vi "Fetch Measurements.vi"(8 "error in (no error)":errorcluster, 11 "Scope In":refnum<k15>) -> (0 "error out":errorcluster, 1 "Phase":dbl format="%.2f", 2 "Actual Gain":dbl, 3 "Scope out":refnum<k15>, 5 "wfm":waveform(dbl)[](array[waveform]))   [LabVIEW 2023, in "Bode Plot - PXI.lvlib"]
uses:
  Bode Plot - PXI.lvlib
  <instrlib>/niScope/Controls/niScope timestamp type.ctl
  <instrlib>/niScope/Controls/niScope scalar measurement.ctl
  <instrlib>/niScope/Controls/niScope array measurement.ctl
  <instrlib>/niScope/Controls/niScope clearable measurement.ctl
  <instrlib>/niScope/Acquire/niScope Multi Read WDT.vi
  <instrlib>/niScope/Measurements/niScope Fetch Measurement.vi
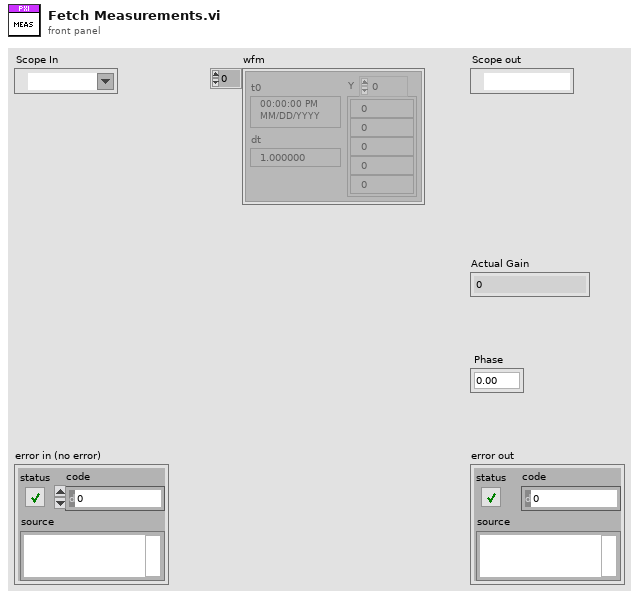
[diagram p1: front panel]
types:
  T1 = typedef "niScope clearable measurement.ctl" = i32
  T2 = typedef "niScope array measurement.ctl" = i32
  T3 = typedef "niScope scalar measurement.ctl" = i32
  T4 = typedef "niScope timestamp type.ctl" = i32
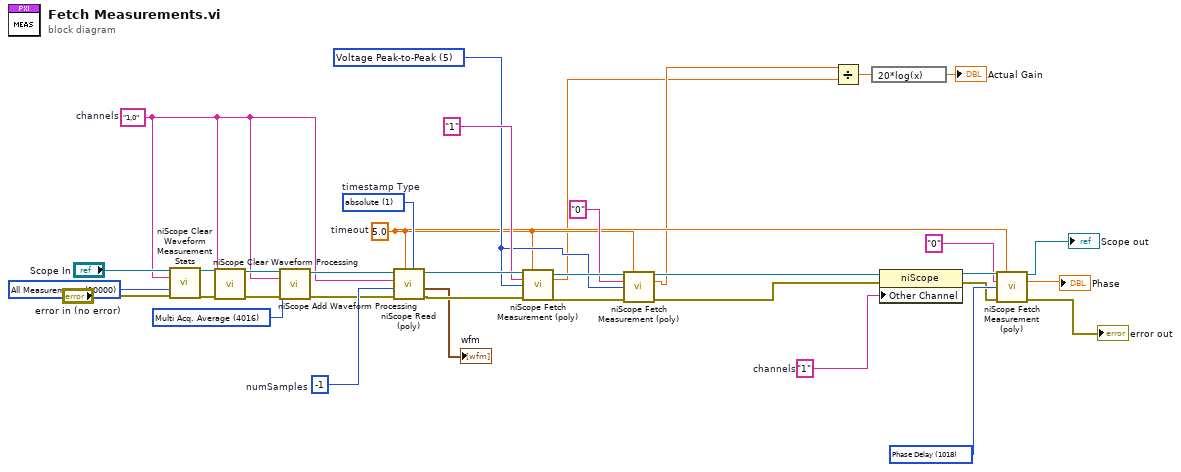
[diagram p0: block diagram]
diagram:
  w5 = T1 10000 items=["All Measurements"=10000, "Multi Acq. Voltage Histogram"=4004, "Multi Acq. Time Histogram"=4005, "Multi Acq. Average"=4016, "Frequency"=2, "Average Frequency"=1016, "FFT Frequency"=1008, "Period"=3, "Average Period"=1015, "Rise Time"=0, "Fall Time"=1, "Rising Slew Rate"=1010, "Falling Slew Rate"=1011, "Overshoot"=18, "Preshoot"=19, "Voltage RMS"=4, "Voltage Cycle RMS"=16, "AC Estimate"=1012, "FFT Amplitude"=1009, "Voltage Average"=10, "Voltage Cycle Average"=17, "DC Estimate"=1013, "Voltage Max"=6, "Voltage Min"=7, "Voltage Peak-to-Peak"=5, "Voltage High"=8, "Voltage Low"=9, "Voltage Amplitude"=15, "Voltage Top"=1007, "Voltage Base"=1006, "Voltage Base-to-Top"=1017, "Negative Width"=11, "Positive Width"=12, "Negative Duty Cycle"=13, "Positive Duty Cycle"=14, "Integral"=1005, "Area"=1003, "Cycle Area"=1004, "Time Delay"=1014, "Phase Delay"=1018, "Low Ref Volts"=1000, "Mid Ref Volts"=1001, "High Ref Volts"=1002, "Volt. Hist. Mean"=2000, "Volt. Hist. Stdev"=2001, "Volt. Hist. Median"=2003, "Volt. Hist. Mode"=2010, "Volt. Hist. Max"=2005, "Volt. Hist. Min"=2006, "Volt. Hist. Peak-to-Peak"=2002, "Volt. Hist. Mean + Stdev"=2007, "Volt. Hist. Mean + 2 Stdev"=2008, "Volt. Hist. Mean + 3 Stdev"=2009, "Volt. Hist. Hits"=2004, "Volt. Hist. New Hits"=2011, "Time Hist. Mean"=3000, "Time Hist. Stdev"=3001, "Time Hist. Median"=3003, "Time Hist. Mode"=3010, "Time Hist. Max"=3005, "Time Hist. Min"=3006, "Time Hist. Peak-to-Peak"=3002, "Time Hist. Mean + Stdev"=3007, "Time Hist. Mean + 2 Stdev"=3008, "Time Hist. Mean + 3 Stdev"=3009, "Time Hist. Hits"=3004, "Time Hist. New Hits"=3011] ("clearable measurement")
  w21 = T2 4016 items=["None"=4000, "Last Acq. Histogram"=4001, "Multi Acq. Voltage Histogram"=4004, "Multi Acq. Time Histogram"=4005, "Multi Acq. Average"=4016, "Polynomial Interpolation"=4011, "Array Integral"=4006, "Derivative"=4007, "Inverse"=4008, "Multiply Channels"=4012, "Add Channels"=4013, "Subtract Channels"=4014, "Divide Channels"=4015, "Array Offset"=4025, "Array Gain"=4026, "Hanning Window"=4009, "Flat Top Window"=4010, "Hamming Window"=4020, "Triangle Window"=4023, "Blackman Window"=4024, "FIR Windowed Filter"=4021, "Bessel IIR Filter"=4022, "Butterworth IIR Filter"=4017, "Chebyshev IIR Filter"=4018, "FFT Phase Spectrum"=4002, "FFT Amp. Spectrum (Volts RMS)"=4003, "FFT Amp. Spectrum (dB)"=4019] ("array measurement")
  w1 = "1,0"  # channels
  w31 = "1"  # channels
  w33 = T3 1018 items=["None"=4000, "Frequency"=2, "Average Frequency"=1016, "FFT Frequency"=1008, "Period"=3, "Average Period"=1015, "Rise Time"=0, "Fall Time"=1, "Rising Slew Rate"=1010, "Falling Slew Rate"=1011, "Overshoot"=18, "Preshoot"=19, "Voltage RMS"=4, "Voltage Cycle RMS"=16, "AC Estimate"=1012, "FFT Amplitude"=1009, "Voltage Average"=10, "Voltage Cycle Average"=17, "DC Estimate"=1013, "Voltage Max"=6, "Voltage Min"=7, "Voltage Peak-to-Peak"=5, "Voltage High"=8, "Voltage Low"=9, "Voltage Amplitude"=15, "Voltage Top"=1007, "Voltage Base"=1006, "Voltage Base-to-Top"=1017, "Negative Width"=11, "Positive Width"=12, "Negative Duty Cycle"=13, "Positive Duty Cycle"=14, "Integral"=1005, "Area"=1003, "Cycle Area"=1004, "Time Delay"=1014, "Phase Delay"=1018, "Low Ref Volts"=1000, "Mid Ref Volts"=1001, "High Ref Volts"=1002, "Volt. Hist. Mean"=2000, "Volt. Hist. Stdev"=2001, "Volt. Hist. Median"=2003, "Volt. Hist. Mode"=2010, "Volt. Hist. Max"=2005, "Volt. Hist. Min"=2006, "Volt. Hist. Peak-to-Peak"=2002, "Volt. Hist. Mean + Stdev"=2007, "Volt. Hist. Mean + 2 Stdev"=2008, "Volt. Hist. Mean + 3 Stdev"=2009, "Volt. Hist. Hits"=2004, "Volt. Hist. New Hits"=2011, "Time Hist. Mean"=3000, "Time Hist. Stdev"=3001, "Time Hist. Median"=3003, "Time Hist. Mode"=3010, "Time Hist. Max"=3005, "Time Hist. Min"=3006, "Time Hist. Peak-to-Peak"=3002, "Time Hist. Mean + Stdev"=3007, "Time Hist. Mean + 2 Stdev"=3008, "Time Hist. Mean + 3 Stdev"=3009, "Time Hist. Hits"=3004, "Time Hist. New Hits"=3011] ("scalar measurement")
  w13 = T3 5 items=["None"=4000, "Frequency"=2, "Average Frequency"=1016, "FFT Frequency"=1008, "Period"=3, "Average Period"=1015, "Rise Time"=0, "Fall Time"=1, "Rising Slew Rate"=1010, "Falling Slew Rate"=1011, "Overshoot"=18, "Preshoot"=19, "Voltage RMS"=4, "Voltage Cycle RMS"=16, "AC Estimate"=1012, "FFT Amplitude"=1009, "Voltage Average"=10, "Voltage Cycle Average"=17, "DC Estimate"=1013, "Voltage Max"=6, "Voltage Min"=7, "Voltage Peak-to-Peak"=5, "Voltage High"=8, "Voltage Low"=9, "Voltage Amplitude"=15, "Voltage Top"=1007, "Voltage Base"=1006, "Voltage Base-to-Top"=1017, "Negative Width"=11, "Positive Width"=12, "Negative Duty Cycle"=13, "Positive Duty Cycle"=14, "Integral"=1005, "Area"=1003, "Cycle Area"=1004, "Time Delay"=1014, "Phase Delay"=1018, "Low Ref Volts"=1000, "Mid Ref Volts"=1001, "High Ref Volts"=1002, "Volt. Hist. Mean"=2000, "Volt. Hist. Stdev"=2001, "Volt. Hist. Median"=2003, "Volt. Hist. Mode"=2010, "Volt. Hist. Max"=2005, "Volt. Hist. Min"=2006, "Volt. Hist. Peak-to-Peak"=2002, "Volt. Hist. Mean + Stdev"=2007, "Volt. Hist. Mean + 2 Stdev"=2008, "Volt. Hist. Mean + 3 Stdev"=2009, "Volt. Hist. Hits"=2004, "Volt. Hist. New Hits"=2011, "Time Hist. Mean"=3000, "Time Hist. Stdev"=3001, "Time Hist. Median"=3003, "Time Hist. Mode"=3010, "Time Hist. Max"=3005, "Time Hist. Min"=3006, "Time Hist. Peak-to-Peak"=3002, "Time Hist. Mean + Stdev"=3007, "Time Hist. Mean + 2 Stdev"=3008, "Time Hist. Mean + 3 Stdev"=3009, "Time Hist. Hits"=3004, "Time Hist. New Hits"=3011] ("scalar measurement")
  w35 = T4 1 items=["relative", "absolute"]  # timestamp Type
  w11 = 5.0  # timeout
  w36 = -1  # numSamples
  n1 = call <instrlib>:"niScope Clear Waveform Measurement Stats.vi"("instrument handle"="Scope In", "channels"=w1, "clearable measurement"=w5, "error in"="error in (no error)") -> ("instrument handle out"=w4:refnum<k15>, "error out"=w3:errorcluster)  [unwired: 10 in]
  n2 = call <instrlib>:"niScope Clear Waveform Processing.vi"("instrument handle"=w4, "channels"=w1, "error in"=w3) -> ("instrument handle out"=w19:refnum<k15>, "error out"=w20:errorcluster)  [unwired: 11 in]
  n3 = call <instrlib>:"niScope Add Waveform Processing.vi"("instrument handle"=w19, "channels"=w1, "array measurement"=w21, "error in"=w20) -> ("instrument handle out"=w17:refnum<k15>, "error out"=w18:errorcluster)  [unwired: 10 in]
  n4 = call-poly <instrlib>:"niScope Read (poly).vi"("timestamp Type"=w35, "timeout"=w11, "error in"=w18, "numSamples"=w36, "channels"=w1, "instrument handle"=w17) -> ("error out"=w32:errorcluster, "wfm"=→"wfm":waveform(dbl)[], "instrument handle out"=w34:refnum<k15>)  [unwired: 2 in, 1 out]
  n5 = call-poly <instrlib>:"niScope Fetch Measurement (poly).vi"("instrument handle"=w34, "timeout"=w11, "channels"="1", "scalar measurement"=w13, "error in"=w32) -> ("instrument handle out"=w15:refnum<k15>, "result"=w8:dbl, "error out"=w12:errorcluster)  [unwired: 8 in]
  n6 = call-poly <instrlib>:"niScope Fetch Measurement (poly).vi"("instrument handle"=w15, "timeout"=w11, "channels"="0", "scalar measurement"=w13, "error in"=w12) -> ("instrument handle out"=w10:refnum<k15>, "result"=w9:dbl, "error out"=w2:errorcluster)  [unwired: 8 in]
  n7 = Divide(x=w9, y=w8) -> (x/y=w30:dbl)
  n8 = expression code="20*log(x)"(w30) -> (→"Actual Gain":dbl)
  n9 = property class="niScope"(reference=w10, error in=w2, "Other Channel"=w31) -> (reference out=w28:refnum<k15>, error out=w27:errorcluster)
  n10 = call-poly <instrlib>:"niScope Fetch Measurement (poly).vi"("instrument handle"=w28, "timeout"=w11, "channels"="0", "scalar measurement"=w33, "error in"=w27) -> ("instrument handle out"=→"Scope out":refnum<k15>, "result"=→"Phase":dbl, "error out"=→"error out":errorcluster)  [unwired: 8 in]
